vi "Copy_Web_Server_File.vi"(8 "error in (no error)":errorcluster, 10 "preview only?":bool, 11 "AB_Application in":refnum<class "AB_Application.lvclass">) -> (0 "error out":errorcluster, 1 "copied web server files":path[](array[path]), 2 "copiedFileGUIDs":string[](array[string]), 3 "AB_Application out":refnum<class "AB_Application.lvclass">)   [LabVIEW 2020, in "AB_Application.lvclass"]
uses:
  <vilib>/AppBuilder/AB_Classes/Application/AB_Application.lvclass
  e:/builds/penguin/labview/branches/2020/dev/dist/vi.lib/AppBuilder/AB_Classes/Build/AB_Build.lvclass
  e:/builds/penguin/labview/branches/2020/dev/dist/vi.lib/AppBuilder/AB_Classes/TargetFile/AB_Targetfile.lvclass
  <vilib>/AppBuilder/AB_Classes/TargetFile/AB_Targetfile.lvclass
  <vilib>/AppBuilder/AB_Classes/Build/AB_Build.lvclass
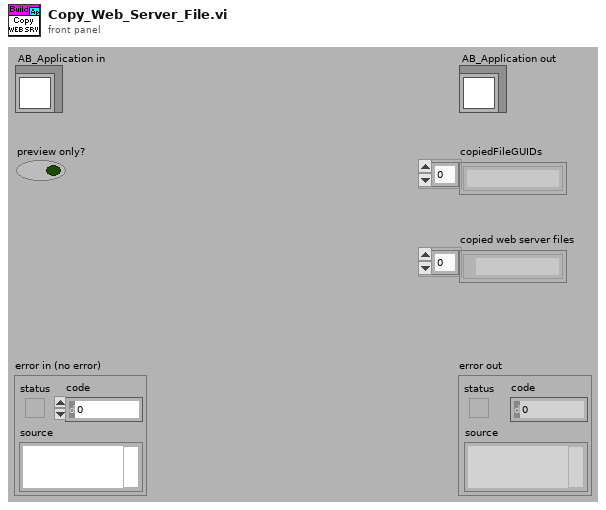
[diagram p1: front panel]
types:
  T1 = typedef "AB_Build.ctl" = cluster{"buildSpecName":string, "buildSpecDescription":string, "destinations":refnum<class "AB_Destination.lvclass">[], "exclusionOption":T2, "defaultLanguage":string, "supportedLanguages":string[], "excludedDirectories":path[], "buildContext":refnum<vi>, "buildObject":T3, "preview":bool, "programatic":bool, "progressBarEvents":T4, "userLog_Path":path, "preActionID":string, "preAction_Path":path, "postActionID":string, "postAction_Path":path, "eng_checkForBrokenVIs?":bool, "eng_verboseLinkerErrors?":bool, "localDest_Path":path, "targetDest_Path":path, "removeVIObject":u16, "cache":refnum<class "PreviewCache.lvclass">, "use cache":bool, "previewCache_ID":string, "buildCache_ID":string, "eng_TempLocalDest_Path":path, "eng_collectDependencies?":bool, "versionInfo":cluster{"buildVersion":cluster{"major":u16, "minor":u16, "patch":u16, "build":u16}, "autoIncrement":bool}, "eng_enableVIChecksums":bool}
  T2 = typedef "AB_Exclusion_Option.ctl" = cluster{"typedefs":bool, "polymorphicVIs":bool, "unusedLibraryItems":bool, "modifyLibraryFile":bool, "edit-timeDependencies":bool, "inlineVIs":bool, "dependent PPLs":bool, "dependent DLLs":bool}
  T3 = typedef "ItemRef.ctl" = u64
  T4 = typedef "provcom_ProgressBar_Events.ctl" = cluster{"newJob":refnum<user-event>, "newItem":refnum<user-event>, "errorMsg":T5, "cancel":refnum<user-event>}
  T5 = typedef "mxLvBuildError.ctl" = refnum<user-event>
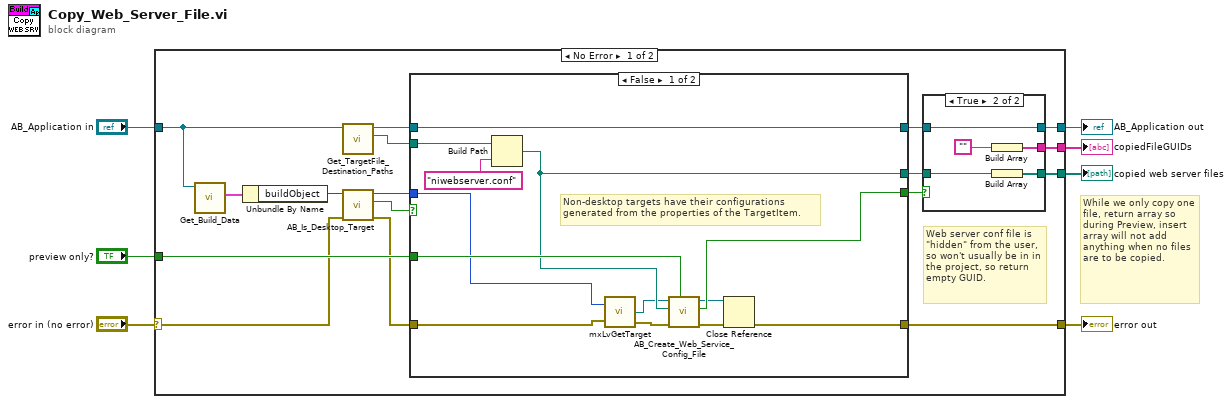
[diagram p0: block diagram]
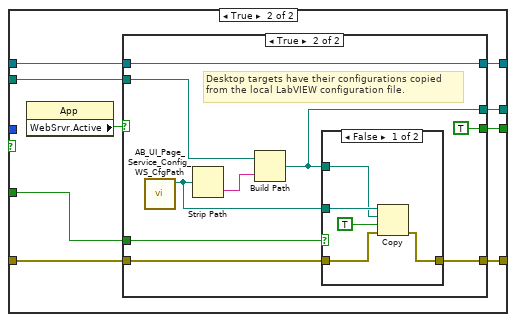
[diagram p3: hidden frame]
diagram:
  # "While we only copy one file, return array so during Preview, insert array will not add anything when no files are to be copied."
  n1 = case shown="No Error" "error in (no error)" {
    selector: "error in (no error)" -> [w21 w71]
    tunnel: [w20 w71] -> w6
    tunnel: [w12 w70] -> w4
    tunnel: "AB_Application in" -> [w17 w70]
    tunnel: "preview only?" -> [w24 _]
    tunnel: [w14 _] -> w1
    tunnel: [w13 _] -> w2
    frame No Error {
      # "Web server conf file is \"hidden\" from the user, so won't usually be in in the project, so return empty GUID."
      n2 = call <vilib>:"Get_Build_Data.vi"("Class in"=w17) -> ("data"=w23:T1)  [unwired: 8 in, 2 out]
      n3 = Unbundle By Name(w23) -> ("buildObject"=w22:T3)
      n4 = call <vilib>:"Get_TargetFile_Destination_Paths.vi"("AB_Targetfile in"=w17) -> ("destination path"=w15:path, "AB_Targetfile out"=w16:refnum<class "AB_Application.lvclass">)  [unwired: 6 in, 3 out]
      n5 = call <resource>:"AB_Is_Desktop_Target.vi"("error in (no error)"=w21, "Object"=w22) -> ("error out"=w19:errorcluster, "Desktop target"=w18:bool, "Object"=w8:T3)  [unwired: 7 in]
      n6 = case shown="False" w18 {
        tunnel: w24 -> [w39 w52]
        tunnel: [w37 w51] -> w10
        tunnel: w16 -> [w37 w49]
        tunnel: [w40 w48] -> w20
        tunnel: w19 -> [w41 w47]
        tunnel: w15 -> [w43 w46]
        tunnel: [w38 w44] -> w11
        tunnel: [w36 w45] -> w9
        tunnel: w8 -> [w35 _]
        frame False {
          # "Non-desktop targets have their configurations\ngenerated from the properties of the TargetItem."
          n7 = Build Path(base path=w43, name or relative path="niwebserver.conf") -> (appended path=w36:path)
          n8 = call <resource>:"mxLvGetTarget.vi"("Item"=w35, "error in"=w41) -> ("Target"=w34:refnum<vi>, "error out"=w33:errorcluster)  [unwired: 1 out]
          n9 = call <resource>:"AB_Create_Web_Service_Config_File.vi"("preview only?"=w39, "error in (no error)"=w33, "path to output configuration"=w36, "target refnum in"=w34) -> ("error out"=w32:errorcluster, "generated?"=w38:bool, "target refnum out"=w31:refnum<vi>)  [unwired: 5 in]
          n10 = Close Reference(reference=w31, error in (no error)=w32) -> (error out=w40:errorcluster)
        }
        frame True {
          n11 = property class="App"() -> ("WebSrvr.Active"=w50:bool)  [unwired: 2 in, 2 out]
          n12 = case shown="True" w50 {
            tunnel: w52 -> [_ w62]
            tunnel: w49 -> [w54 w58]
            tunnel: [w54 w58] -> w51
            tunnel: w47 -> [w53 w61]
            tunnel: [w53 w60] -> w48
            tunnel: [_ w56] -> w45
            tunnel: w46 -> [_ w57]
            tunnel: [_ TRUE] -> w44
            frame False {
              # "If web server is not enabled, there is no need to copy anything."
            }
            frame True {
              # "Desktop targets have their configurations copied\nfrom the local LabVIEW configuration file."
              n13 = call <resource>:"AB_UI_Page_Service_Config_WS_CfgPath.vi"() -> ("config file"=w63:path)  [unwired: 10 in, 1 out]
              n14 = Strip Path(path=w63) -> (name=w59:string)  [unwired: 1 out]
              n15 = Build Path(base path=w57, name or relative path=w59) -> (appended path=w56:path)
              n16 = case shown="False" w62 {
                tunnel: w63 -> [w68 _]
                tunnel: w56 -> [w67 _]
                tunnel: w61 -> [w65 w69]
                tunnel: [w64 w69] -> w60
                frame False {
                  n17 = Copy(8:w65, 9:TRUE ("overwrite (F)"), 10:w67, 11:w68) -> (0:w64:errorcluster)  [unwired: 1 in, 2 out]
                }
                frame True {
                }
              }
            }
          }
        }
      }
      n18 = case shown="True" w11 {
        tunnel: [_ w29] -> w14
        tunnel: [_ w28] -> w13
        tunnel: w10 -> [w25 w27]
        tunnel: [w25 w27] -> w12
        tunnel: w9 -> [_ w26]
        frame False {
        }
        frame True {
          n19 = Build Array("") -> (w29:string[])
          n20 = Build Array(w26) -> (w28:path[])
        }
      }
    }
    frame Error {
    }
  }
  "error out" <- w6
  "AB_Application out" <- w4
  "copied web server files" <- w2
  "copiedFileGUIDs" <- w1
